vi "Hardware Config.vi"() -> ()   [LabVIEW 2022 SP3]
uses:
  Controls/Config..ctl
panel:
  in  "Power 2":bool
  in  "Load Configuration":bool
  in  "New configuration":bool
  in  "Save Config":bool
  in  "Tab Control":enum32{"DO", "AI", "AI PROPLUSION"}(tab)
  in  "DO  Configuration":T1(array[cluster])=[{"NAME"="GD COM", "lines"="cDAQ1Mod2_1/port0/line0", "Default_Value"=FALSE, "DO invert?"=FALSE}, {"NAME"="Motor Command", "lines"="cDAQ1Mod2_1/port0/line1", "Default_Value"=FALSE, "DO invert?"=FALSE}]
  in  "AI Config":T2(array[cluster])
  in  "AI Config 2":T2(array[cluster])
  # "D.S.C.CHARUDATTA"
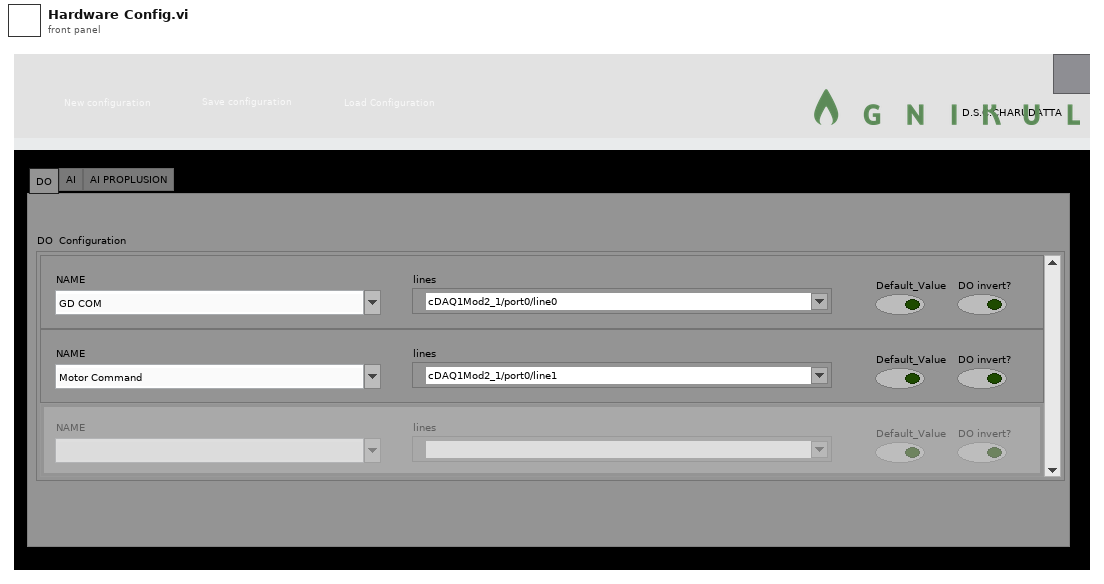
[diagram p1: front panel]
types:
  T1 = cluster{"NAME":string, "lines":tag, "Default_Value":bool, "DO invert?":bool}[]
  T2 = cluster{"AI signal Lists":string, "AI Channel List":tag, "Prescale Min":dbl, "Prescale Max":dbl, "Sensor Min":dbl, "Sensor Max":dbl, "Units":string}[]
  T3 = typedef "Config..ctl" = cluster{"AO config":cluster{"Channel_Name":string, "Channel_Number":string, "Default_Value":dbl, "Units":string}[], "AI config":cluster{"Channel_Name":string, "Channel_Number":string, "Pre_Scale_min":dbl, "Pre_Scale_max":dbl, "Sensor_min":dbl, "Sensor_max":dbl, "Units":string}[], "DI config":cluster{"Channel_Name":string, "Channel_Number":string, "Default_Value":bool, "DI invert?":bool}[], "DO config":cluster{"Channel_Name":string, "Channel_Number":string, "Default_Value":bool, "DO invert?":bool}[], "TC config":cluster{"Channel_Name":string, "Channel_Number":string, "Pre_Scale_min":dbl, "Pre_Scale_max":dbl, "units":i32, " type":i32}[], "ACC config":cluster{"Channel_Name":string, "Channel_Number":string, "Pre_Scale_min":dbl, "Pre_Scale_max":dbl, "Terminal configuration":i32, "Sensitivity":dbl, "Sensitivity units":i32}[], "SG config":cluster{"Channel_Name":string, "Channel_Number":string, "Pre_Scale_min":dbl, "Pre_Scale_max":dbl}[], "Strain Gauge Settings":cluster{"poisson ratio":dbl, "nominal gage resistance":dbl, "gage factor":dbl}, "Bridge Settings":cluster{"voltage excitation value":dbl, "voltage excitation source":i32, "initial bridge voltage":dbl, "lead wire resistance":dbl, "strain configuration":i32}, "Sample Rate":cluster{"AI Sample Rate":dbl[], "AO Sample Rate":dbl[], "DI Sample Rate":dbl[], "TC Sample Rate":dbl[], "DO Sample Rate":dbl[], "SG Sample Rate":dbl[], "ACC Sample Rate":dbl[]}, "AI PROPLUSION":cluster{"Channel_Name":string, "Channel_Number":string, "Pre_Scale_min":dbl, "Pre_Scale_max":dbl, "Sensor_min":dbl, "Sensor_max":dbl, "Units":string}[]}
  T4 = enum16{"open", "replace", "create", "open or create", "replace or create", "replace or create with confirmation"}
  T5 = cluster{"Data":T3, "path":path, "Name ref":refnum<vi>[], "Names":string[][], "Signal path":path, "SR":cluster{"AI Sample Rate":dbl[], "AO Sample Rate":dbl[], "DI Sample Rate":dbl[], "TC Sample Rate":dbl[], "DO Sample Rate":dbl[], "SG Sample Rate":dbl[], "ACC Sample Rate":dbl[]}, "Device List":cluster{"AO Cards":tag[], "AI Cards":tag[], "DI Cards":tag[], "DO Cards":tag[]}}
  T6 = cluster{"Channel_Name":string, "Channel_Number":string, "Default_Value":bool, "DO invert?":bool}[]
  T7 = cluster{"Channel_Name":string, "Channel_Number":string, "Pre_Scale_min":dbl, "Pre_Scale_max":dbl, "Sensor_min":dbl, "Sensor_max":dbl, "Units":string}[]
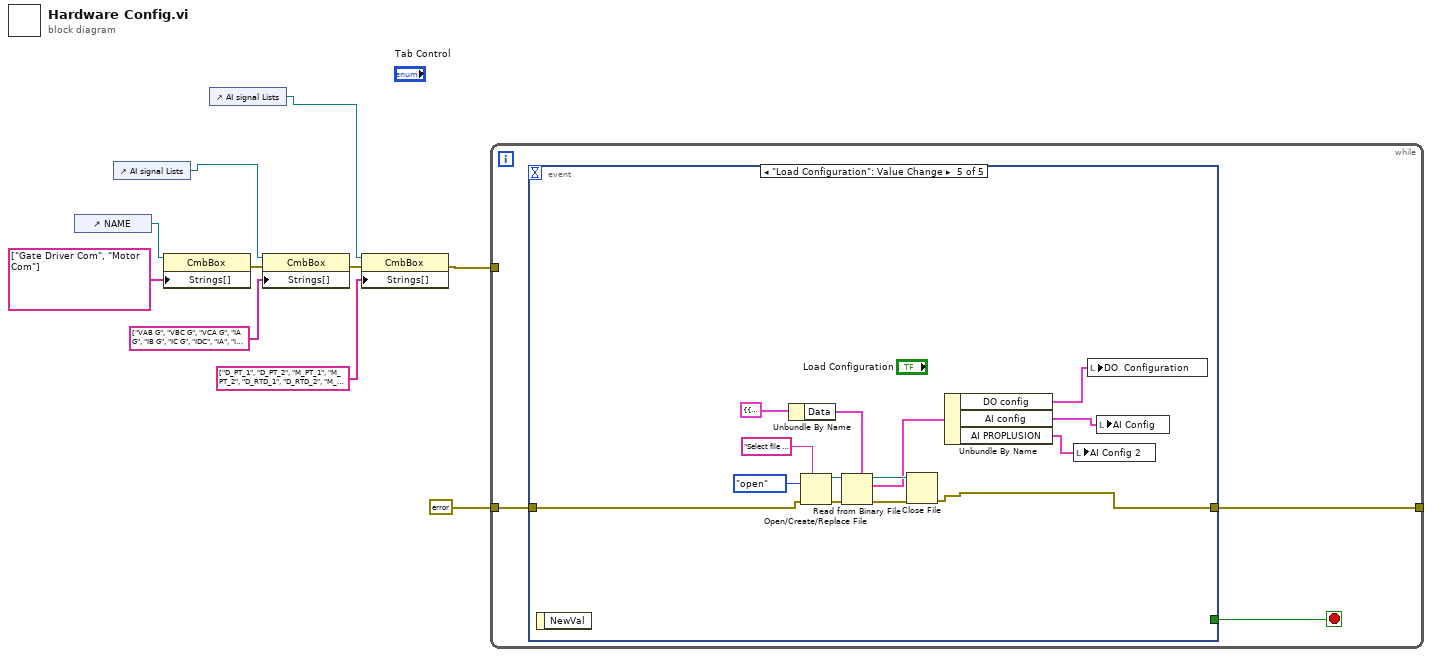
[diagram p0: block diagram]
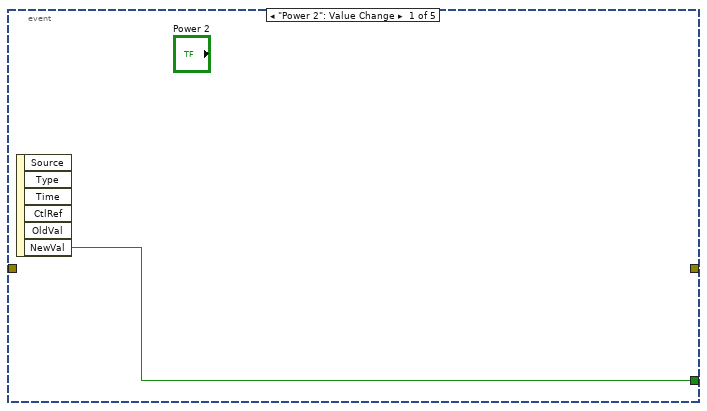
[diagram p2: hidden frame]
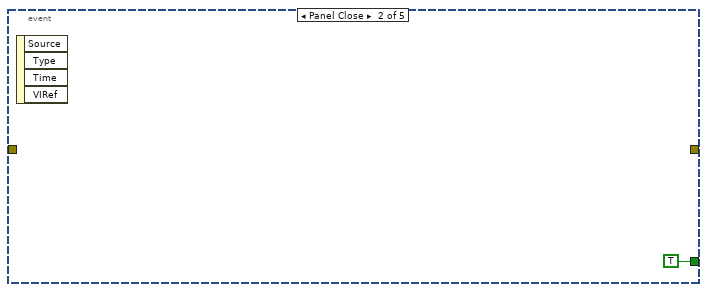
[diagram p3: hidden frame]
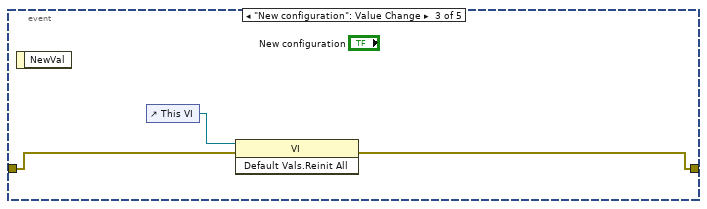
[diagram p4: hidden frame]
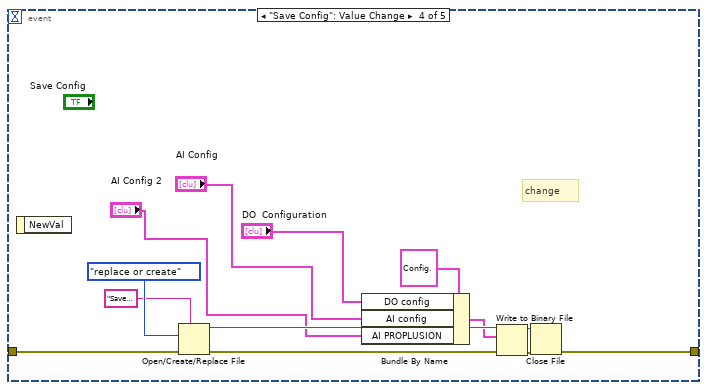
[diagram p5: hidden frame]
diagram:
  n1 = control-ref of="NAME"() -> (w8:refnum<vi>)
  n2 = control-ref of="AI signal Lists"() -> (w1:refnum<vi>)
  n3 = property class="CmbBox"(reference=w8, "Strings[]"=string[] ["Gate Driver Com", "Motor Com"] ("channel name(s) in (Untitled)")) -> (error out=w5:errorcluster)  [unwired: 1 in, 1 out]
  n4 = control-ref of="AI signal Lists"() -> (w2:refnum<vi>)
  n5 = property class="CmbBox"(reference=w1, error in=w5, "Strings[]"=string[] ["VAB G", "VBC G", "VCA G", "IA G", "IB G", "IC G", "IDC", "IA", "IB", "IC", "IDC_G", "VAB", "VBC", "VCA", "VDC_G", "VDC"] ("channel name(s) in (Untitled)")) -> (error out=w4:errorcluster)  [unwired: 1 out]
  n6 = property class="CmbBox"(reference=w2, error in=w4, "Strings[]"=string[] ["D_PT_1", "D_PT_2", "M_PT_1", "M_PT_2", "D_RTD_1", "D_RTD_2", "M_RTD_1", "M_RTD_2", "M_RTD_3", "M_PT_3"] ("channel name(s) in (Untitled)")) -> (error out=w3:errorcluster)  [unwired: 1 out]
  n7 = while {
    tunnel: [w12] -> _
    tunnel: errorcluster {"status"=FALSE, "code"=0, "source"=""} ("error in") -> [w11]
    tunnel: w3 -> [_]
    stop <- w13 stop-if-true
    n8 = event shown="[4] \"Load Configuration\": Value Change" {
      selector: _ -> [_ _ _ _ _]
      dyn-events: _ -> [_ _ _ _ _]
      timeout: _ -> [_ _ _ _ _]
      tunnel: [w14 TRUE ("NewVal") _ _ _] -> w13
      tunnel: [_ _ w17 w29 w38] -> w12
      tunnel: w11 -> [_ _ w18 w21 w37]
      event "Power 2": Value Change {
        n9 = event-data() -> ("NewVal"=w14:bool)  [unwired: 1 in, 5 out]
      }
      event Panel Close {
        n10 = event-data() -> ()  [unwired: 1 in, 4 out]
      }
      event "New configuration": Value Change {
        n11 = event-data() -> ()  [unwired: 1 in, 1 out]
        n12 = control-ref of="This VI"() -> (w16:refnum<vi>)
        n13 = invoke class="VI" method="Default Vals.Reinit All"(reference=w16, error in=w18) -> (error out=w17:errorcluster)  [unwired: 1 in, 2 out]
      }
      event "Save Config": Value Change {
        # "change"
        n14 = event-data() -> ()  [unwired: 1 in, 1 out]
        n15 = Open/Create/Replace File(error in=w21, prompt="Save Changes", operation (0:open)=T4."replace or create") -> (refnum out=w28:refnum<file>, error out=w22:errorcluster)  [unwired: 3 in, 1 out]
        n16 = Bundle By Name(cluster=T3 {"AO config"=[], "AI config"=[], "DI config"=[], "DO config"=[], "TC config"=[{"Channel_Name"="", "Channel_Number"="", "Pre_Scale_min"=0.0, "Pre_Scale_max"=0.0, "units"=4, " type"=7}], "ACC config"=[], "SG config"=[], "Strain Gauge Settings"={"poisson ratio"=0.3, "nominal gage resistance"=120.0, "gage factor"=2.08}, "Bridge Settings"={"voltage excitation value"=3.3, "voltage excitation source"=10200, "initial bridge voltage"=0.0, "lead wire resistance"=1.7, "strain configuration"=10271}, "Sample Rate"={"AI Sample Rate"=[], "AO Sample Rate"=[], "DI Sample Rate"=[], "TC Sample Rate"=[], "DO Sample Rate"=[], "SG Sample Rate"=[], "ACC Sample Rate"=[]}, "AI PROPLUSION"=[]} ("Data"), "DO config"="DO  Configuration", "AI config"="AI Config", "AI PROPLUSION"="AI Config 2") -> (w24:T3)
        n17 = Write to Binary File(file (use dialog)=w28, data=w24, error in=w22) -> (refnum out=w31:refnum<file>, error out=w30:errorcluster)  [unwired: 3 in, 1 out]
        n18 = Close File(refnum=w31, error in=w30) -> (error out=w29:errorcluster)  [unwired: 1 out]
      }
      event "Load Configuration": Value Change {
        n19 = event-data() -> ()  [unwired: 1 in, 1 out]
        n20 = Unbundle By Name(T5 {"Data"={"AO config"=[], "AI config"=[], "DI config"=[], "DO config"=[], "TC config"=[], "ACC config"=[], "SG config"=[], "Strain Gauge Settings"={"poisson ratio"=0.0, "nominal gage resistance"=0.0, "gage factor"=0.0}, "Bridge Settings"={"voltage excitation value"=0.0, "voltage excitation source"=0, "initial bridge voltage"=0.0, "lead wire resistance"=0.0, "strain configuration"=0}, "Sample Rate"={"AI Sample Rate"=[], "AO Sample Rate"=[], "DI Sample Rate"=[], "TC Sample Rate"=[], "DO Sample Rate"=[], "SG Sample Rate"=[], "ACC Sample Rate"=[]}, "AI PROPLUSION"=[]}, "path"=path "", "Name ref"=[], "Names"=[], "Signal path"=path "", "SR"={"AI Sample Rate"=[], "AO Sample Rate"=[], "DI Sample Rate"=[], "TC Sample Rate"=[], "DO Sample Rate"=[], "SG Sample Rate"=[], "ACC Sample Rate"=[]}, "Device List"={"AO Cards"=[], "AI Cards"=[], "DI Cards"=[], "DO Cards"=[]}} ("input cluster")) -> ("Data"=w39:T3)
        n21 = Open/Create/Replace File(error in=w37, prompt="Select file to load", operation (0:open)=T4."open") -> (refnum out=w42:refnum<file>, error out=w45:errorcluster)  [unwired: 3 in, 1 out]
        n22 = Read from Binary File(5:w39, 8:w45, 11:w42) -> (0:w43:errorcluster, 2:w35:T3, 3:w44:refnum<file>)  [unwired: 3 in, 1 out]
        n23 = Close File(refnum=w44, error in=w43) -> (error out=w38:errorcluster)  [unwired: 1 out]
        n24 = Unbundle By Name(w35) -> ("DO config"=w34:T6, "AI config"=w33:T7, "AI PROPLUSION"=w32:T7)
        n25 = local write "AI Config 2"(w32) -> ()
        n26 = local write "DO  Configuration"(w34) -> ()
        n27 = local write "AI Config"(w33) -> ()
      }
    }
  }
